vi "Template - Scope Transfer Current Waveform.vi"() -> ()   [LabVIEW 2020]
doc: "This example shows how to transfer the current waveform on an oscilloscope. Users can setup the acquired waveform using the instrument's front panel interface and then transfer that waveform to the computer using this example."
uses:
  <instrlib>/_Template - Scope/Template - Scope.lvlib
panel:
  in  "Serial Configuration":T1={"Baud Rate"=9600, "Parity"=0, "Data Bits"=7, "Stop Bits"=10, "Flow Control"=0} {"Flow Control" items=["None", "XON/XOFF", "RTS/CTS", "XON/XOFF & RTS/CTS", "DTR/DSR", "XON/XOFF & DTR/DSR"]; "Stop Bits" items=["1.0"=10, "1.5"=15, "2.0"=20]; "Data Bits" items=["7"=7, "8"=8]; "Parity" items=["None", "Odd", "Even", "Mark", "Space"]; "Baud Rate" items=["300"=300, "600"=600, "1200"=1200, "2400"=2400, "4800"=4800, "9600"=9600, "19200"=19200]}
  in  "Timeout (10000 ms)":u32=10000
  out "Waveform Data":waveform(dbl)(graph)
  in  "Channel (1: Channel 1)":u16(ring)=1 items=["Channel 1"=1, "Channel 2"=2]
  in  "VISA resource name":refnum<visa-resource-name>
  # "(c) 2014 <Enter Company Name Here>.  ALL RIGHTS RESERVED."
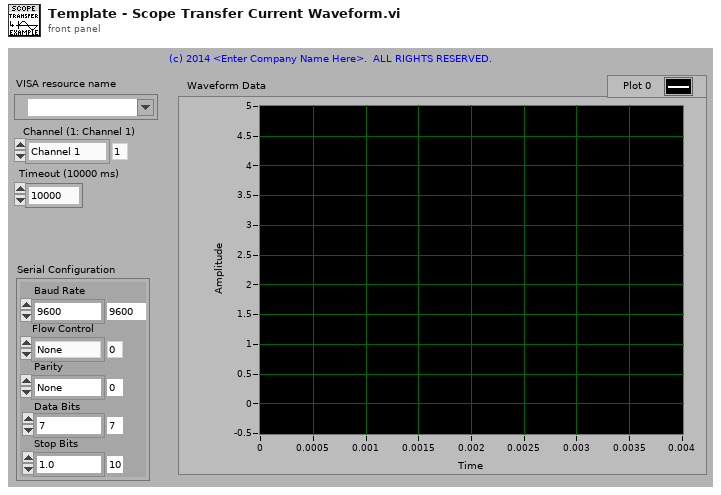
[diagram p1: front panel]
types:
  T1 = cluster{"Baud Rate":u32, "Parity":u16, "Data Bits":u16, "Stop Bits":u16, "Flow Control":u16}
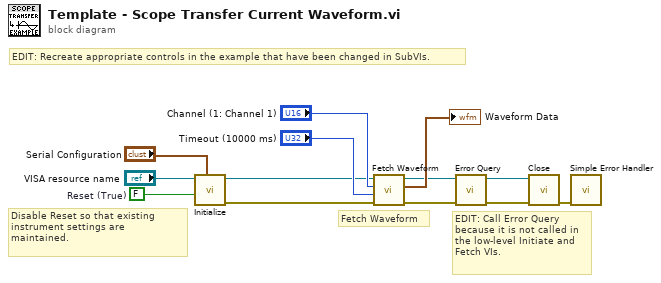
[diagram p0: block diagram]
diagram:
  w1 = FALSE  # Reset (True)
  # "EDIT: Call Error Query because it is not called in the low-level Initiate and Fetch VIs."
  # "EDIT: Recreate appropriate controls in the example that have been changed in SubVIs."
  # "Disable Reset so that existing instrument settings are maintained."
  # "Fetch Waveform"
  n1 = call <instrlib>:"Initialize.vi"("Serial Configuration"="Serial Configuration", "Reset (True)"=w1, "VISA resource name"="VISA resource name") -> ("error out"=w7:errorcluster, "VISA resource name out"=w8:refnum<visa-resource-name>)  [unwired: 7 in]
  n2 = call <instrlib>:"Fetch Waveform.vi"("error in (no error)"=w7, "Timeout (10000 ms)"="Timeout (10000 ms)", "Channel (1: Channel 1)"="Channel (1: Channel 1)", "VISA resource name"=w8) -> ("error out"=w3:errorcluster, "Waveform Data"=→"Waveform Data":waveform(dbl), "VISA resource name out"=w5:refnum<visa-resource-name>)  [unwired: 5 in]
  n3 = call <instrlib>:"Error Query.vi"("error in (no error)"=w3, "VISA resource name"=w5) -> ("error out"=w2:errorcluster, "VISA resource name out"=w4:refnum<visa-resource-name>)  [unwired: 6 in, 2 out]
  n4 = call <instrlib>:"Close.vi"("error in (no error)"=w2, "VISA resource name"=w4) -> ("error out"=w13:errorcluster)  [unwired: 9 in]
  n5 = call <vilib>:"Simple Error Handler.vi"("error in (no error)"=w13) -> ()  [unwired: 4 in, 5 out]
